vi "Configure Pseudo Card.vi"(8 "error in (no error)":errorcluster, 9 "Slot Number (0: slot1)":i32(ring) items=["slot 1", "slot 2"], 10 "Pseudo Card (0:No pseudocard)":i32(ring) items=["0", "7700", "7701", "7702", "7703", "7705", "7706", "7707", "7708", "7709", "7710", "7711", "7712"], 11 "VISA resource name":refnum<visa-resource-name>) -> (0 "error out":errorcluster, 3 "VISA resource name out":refnum<visa-resource-name>)   [LabVIEW 2024, in "Keithley DMM6500 DAQ6500 Series.lvlib"]
doc: "Specifies a pseudocard to implement for the designated slot.\n\nPseudocards allow you to configure your system without having an actual module installed in your system. You can perform open, close, and scan operations and configure your system with pseudocards.\nThis command is only applicable to slots that do not have a module or pseudocard installed. If a pseudocard is presently assigned to the slot, you must set the slot to no pseudocard before assigning the new pseudocard.\nAfter assigning a pseudocard, you can use valid commands for the module for that slot.\nChanging the pseudocard card assignment from a pseudocard to no pseudocard invalidates scan lists that include that slot."
uses:
  Keithley DMM6500 DAQ6500 Series.lvlib
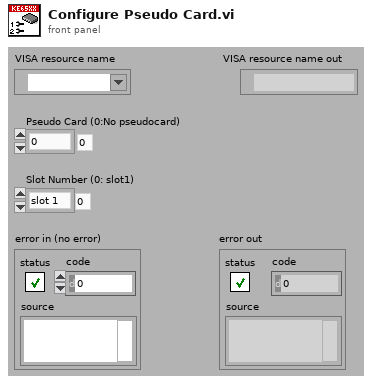
[diagram p1: front panel]
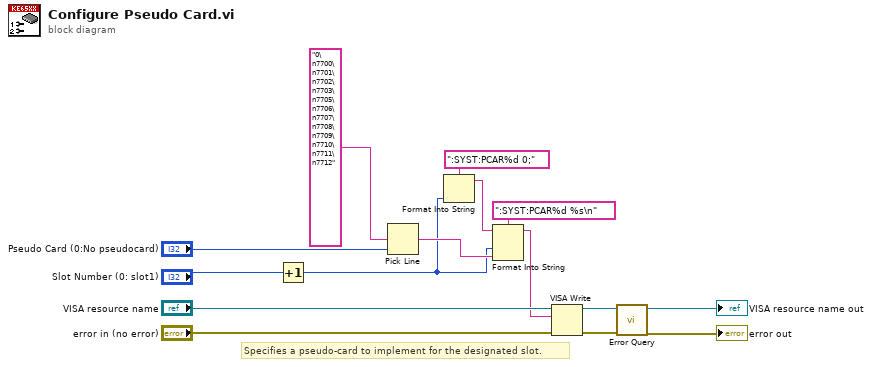
[diagram p0: block diagram]
diagram:
  # "Specifies a pseudo-card to implement for the designated slot."
  n1 = Increment(x="Slot Number (0: slot1)") -> (x+1=w2:i32)
  n2 = Pick Line(multi-line string="0\n7700\n7701\n7702\n7703\n7705\n7706\n7707\n7708\n7709\n7710\n7711\n7712", line index="Pseudo Card (0:No pseudocard)") -> (output string=w5:string)  [unwired: 1 in]
  n3 = Format Into String(format string=":SYST:PCAR%d 0;", w2) -> (resulting string=w4:string)  [unwired: 2 in, 1 out]
  n4 = Format Into String(format string=":SYST:PCAR%d %s\n", initial string=w4, w2, w5) -> (resulting string=w6:string)  [unwired: 1 in, 1 out]
  n5 = VISA Write(VISA resource name="VISA resource name", write buffer=w6, error in (no error)="error in (no error)") -> (VISA resource name out=w13:refnum<visa-resource-name>, error out=w12:errorcluster)  [unwired: 1 out]
  n6 = call "Error Query.vi"("error in (no error)"=w12, "VISA resource name"=w13) -> ("error out"=→"error out":errorcluster, "VISA resource name out"=→"VISA resource name out":refnum<visa-resource-name>)  [unwired: 6 in, 2 out]
